vi "Check In Ref.vi"(8 "error in (no error)":errorcluster, 11 "Ref":refnum<vi>) -> (0 "error out":errorcluster)   [LabVIEW 2015, in "VI.lvlib"]
uses:
  VI.lvlib
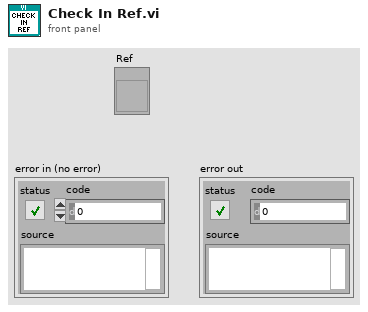
[diagram p1: front panel]
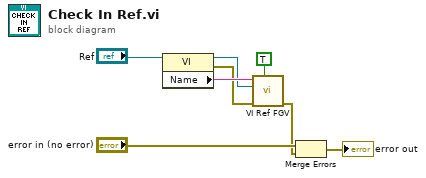
[diagram p0: block diagram]
diagram:
  n1 = property class="VI"(reference="Ref") -> (reference out=w5:refnum<vi>, error out=w2:errorcluster, "Name"=w6:string)  [unwired: 1 in]
  n2 = call "VI Ref FGV.vi"("Check in"=TRUE, "error in (no error)"=w2, "Ref in"=w5, "Name"=w6) -> ("error out"=w3:errorcluster)  [unwired: 5 in, 2 out]
  n3 = Merge Errors("error in (no error)", w3) -> (→"error out":errorcluster)
